vi "Initialize.vi"(8 "error in (no error)":errorcluster, 11 "device data model in":refnum<class "ICPCON PM3114 Data Model.lvclass">) -> (0 "error out":errorcluster, 3 "device data model out":refnum<class "ICPCON PM3114 Data Model.lvclass">)   [LabVIEW 2021, in "ICPCON PM3114 Data Model.lvclass"]
doc: "This VI initializes the device data model."
uses:
  ICPCON PM3114 Data Model.lvclass
  Type Definitions/Data Model.ctl
  ICPCON PM3114 Data Model.lvclass/ICPCON PM3114 Data Model.ctl
  Modbus_v121c/Data Model/Device Data Model.lvclass
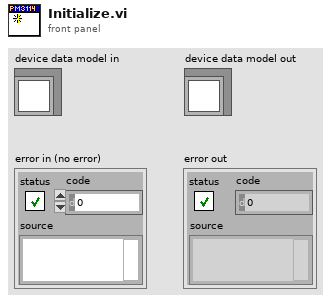
[diagram p1: front panel]
types:
  T1 = typedef "ICPCON PM3114 Data Model.lvclass/Data Model.ctl" = cluster{"UTC":u64, "Power value":sgl[], "ES":u8}
  T2 = typedef "Device Data Model.lvclass/N channel.ctl" = cluster{"N DI channel":i32, "N DO channel":i32, "N AI channel":i32, "N AO channel":i32}
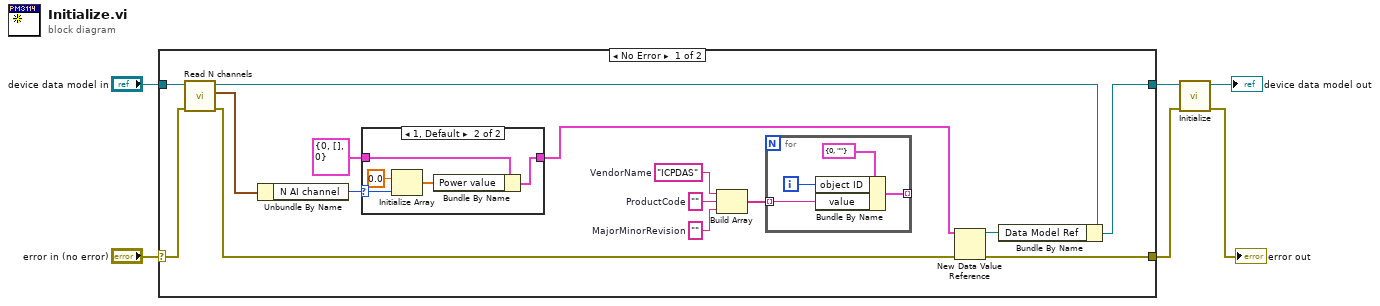
[diagram p0: block diagram]
diagram:
  n1 = case shown="No Error" "error in (no error)" {
    selector: "error in (no error)" -> [w12 w32]
    tunnel: "device data model in" -> [w13 w33]
    tunnel: [w15 w32] -> w5
    tunnel: [w17 w33] -> w4
    frame No Error {
      w19 = ""  # MajorMinorRevision
      w21 = ""  # ProductCode
      w20 = "ICPDAS"  # VendorName
      n2 = call-dynamic "Read N channels.vi"("error in (no error)"=w12, "device data model in"=w13) -> ("error out"=w11:errorcluster, "N channel"=w8:T2, "device data model out"=w14:refnum<class "ICPCON PM3114 Data Model.lvclass">)  [unwired: 7 in]
      n3 = Unbundle By Name(w8) -> ("N AI channel"=w9:i32)
      n4 = case shown="1, Default" w9 {
        selector: w9 -> [_ w23]
        tunnel: T1 {"UTC"=0, "Power value"=[], "ES"=0} ("Data Model") -> [w22 w26]
        tunnel: [w22 w24] -> w7
        frame 0 {
        }
        frame 1, Default {
          n5 = Initialize Array(sgl 0.0 ("Boolean"), w23) -> (w25:sgl[])
          n6 = Bundle By Name(cluster=w26, "Power value"=w25) -> (w24:T1)
        }
      }
      n7 = Build Array(w20, w21, w19) -> (w18:string[])
      n8 = for {
        tunnel: w18 -> [w29] mode=indexing
        tunnel: [w28] -> _ mode=indexing
        i -> [w30]
        n9 = Bundle By Name(cluster=cluster{"object ID":u8, "value":string} {"object ID"=0, "value"=""} ("Cluster"), "object ID"=w30, "value"=w29) -> (w28:cluster{"object ID":u8, "value":string})
      }
      n10 = New Data Value Reference(data value=w7, error in=w11) -> (data value reference=w16:refnum<data-value>, error out=w15:errorcluster)
      n11 = Bundle By Name(cluster=w14, "Data Model Ref"=w16) -> (w17:refnum<class "ICPCON PM3114 Data Model.lvclass">)
    }
    frame Error {
    }
  }
  n12 = call-parent "Initialize.vi"("error in"=w5, "device data model in"=w4) -> ("error out"=→"error out":errorcluster, "device data model out"=→"device data model out":refnum<class "ICPCON PM3114 Data Model.lvclass">)  [unwired: 8 in]
